vi "[CS] [Camera] Get Frame.vi"(8 "size Y":i32, 9 "size X":i32, 10 "size":i64, 11 "buffer in":u8[](array[numeric])) -> (0 "error":bool, 3 "buffer out":u8[][](array[numeric]))   [LabVIEW 2014]
uses:
  <vilib>/Utility/error.llb/DialogType.ctl
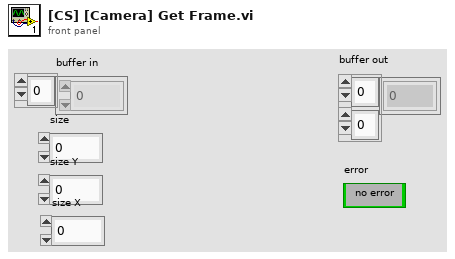
[diagram p1: front panel]
types:
  T1 = typedef "DialogType.ctl" = u16
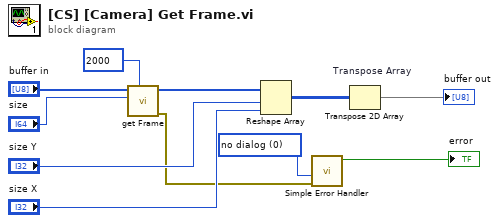
[diagram p0: block diagram]
diagram:
  w2 = T1 0 items=["no dialog", "OK message", "continue or stop message", "OK message + warnings", "continue/stop + warnings"] ("type of dialog (OK msg:1)")
  n1 = call "get Frame.vi"("timeout"=2000, "size"="size", "buffer"="buffer in") -> ("error out"=w3:errorcluster, "buffer out"=w11:u8[])  [unwired: 5 in, 2 out]
  n2 = Reshape Array "Reshape Array"(w11, "size Y", "size X") -> (w8:u8[][])
  n3 = call <vilib>:"Simple Error Handler.vi"("type of dialog (OK msg:1)"=w2, "error in (no error)"=w3) -> ("error?"=→"error":bool)  [unwired: 3 in, 4 out]
  n4 = Transpose 2D Array "Transpose Array"(2D array=w8) -> (transposed array=→"buffer out":u8[][])
